vi "PIDSetpointSet.vi"(4 "Update":bool, 5 "Output Range":cluster{"output high":dbl, "output low":dbl}={"output high"=0.25, "output low"=-0.25}, 6 "Auto":bool, 7 "PID Gains":T1={"proportional gain (Kc)"=1.0, "integral time (Ti, min)"=0.01, "derivative time (Td, min)"=0.0}, 8 "Encoder Position":dbl format="%#_13g", 9 "Level":i8, 10 "Setpoints":dbl[](array[numeric]), 11 "Manual Power":dbl format="%#_13g") -> (0 "Power Out":dbl)   [LabVIEW 2018]
uses:
  <vilib>/addons/control/pid/pid.llb/PID (DBL).vi
  <vilib>/addons/control/pid/NI_PID_pid.lvlib
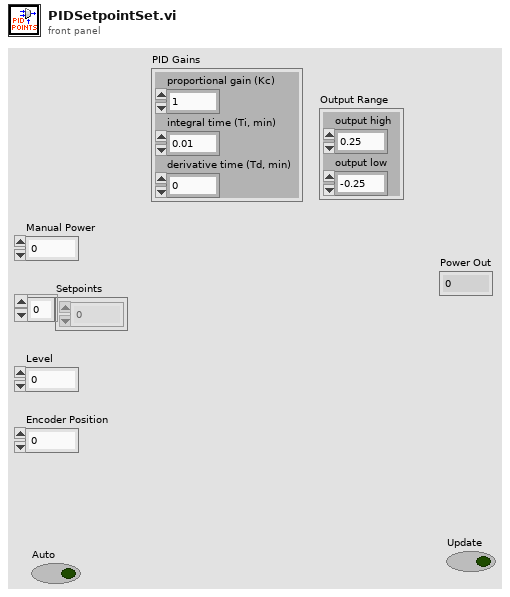
[diagram p1: front panel]
types:
  T1 = cluster{"proportional gain (Kc)":dbl, "integral time (Ti, min)":dbl, "derivative time (Td, min)":dbl}
  T2 = typedef "WPI_SwitchDevRef.ctl" = cluster{"DevStatus":errorcluster, "DIO Channel":T3, "CntIndex":T4, "Normally Closed":bool}
  T3 = typedef "FPGA_DIOChannel.ctl" = enum8{"DIO 0", "DIO 1", "DIO 2", "DIO 3", "DIO 4", "DIO 5", "DIO 6", "DIO 7", "DIO 8", "DIO 9", "DIO MXP 0", "DIO MXP 1", "DIO MXP 2", "DIO MXP 3", "DIO MXP 4", "DIO MXP 5", "DIO MXP 6", "DIO MXP 7", "DIO MXP 8", "DIO MXP 9", "DIO MXP 10", "DIO MXP 11", "DIO MXP 12", "DIO MXP 13", "DIO MXP 14", "DIO MXP 15", "SPI Port CS1", "SPI Port CS2", "SPI Port CS3", "SPI Port MISO", "SPI Port MOSI", "Invalid"}
  T4 = typedef "FPGA_CounterCtrSystemIndex.ctl" = enum8{"Ctr 0", "Ctr 1", "Ctr 2", "Ctr 3", "Ctr 4", "Ctr 5", "Ctr 6", "Ctr 7", "Invalid"}
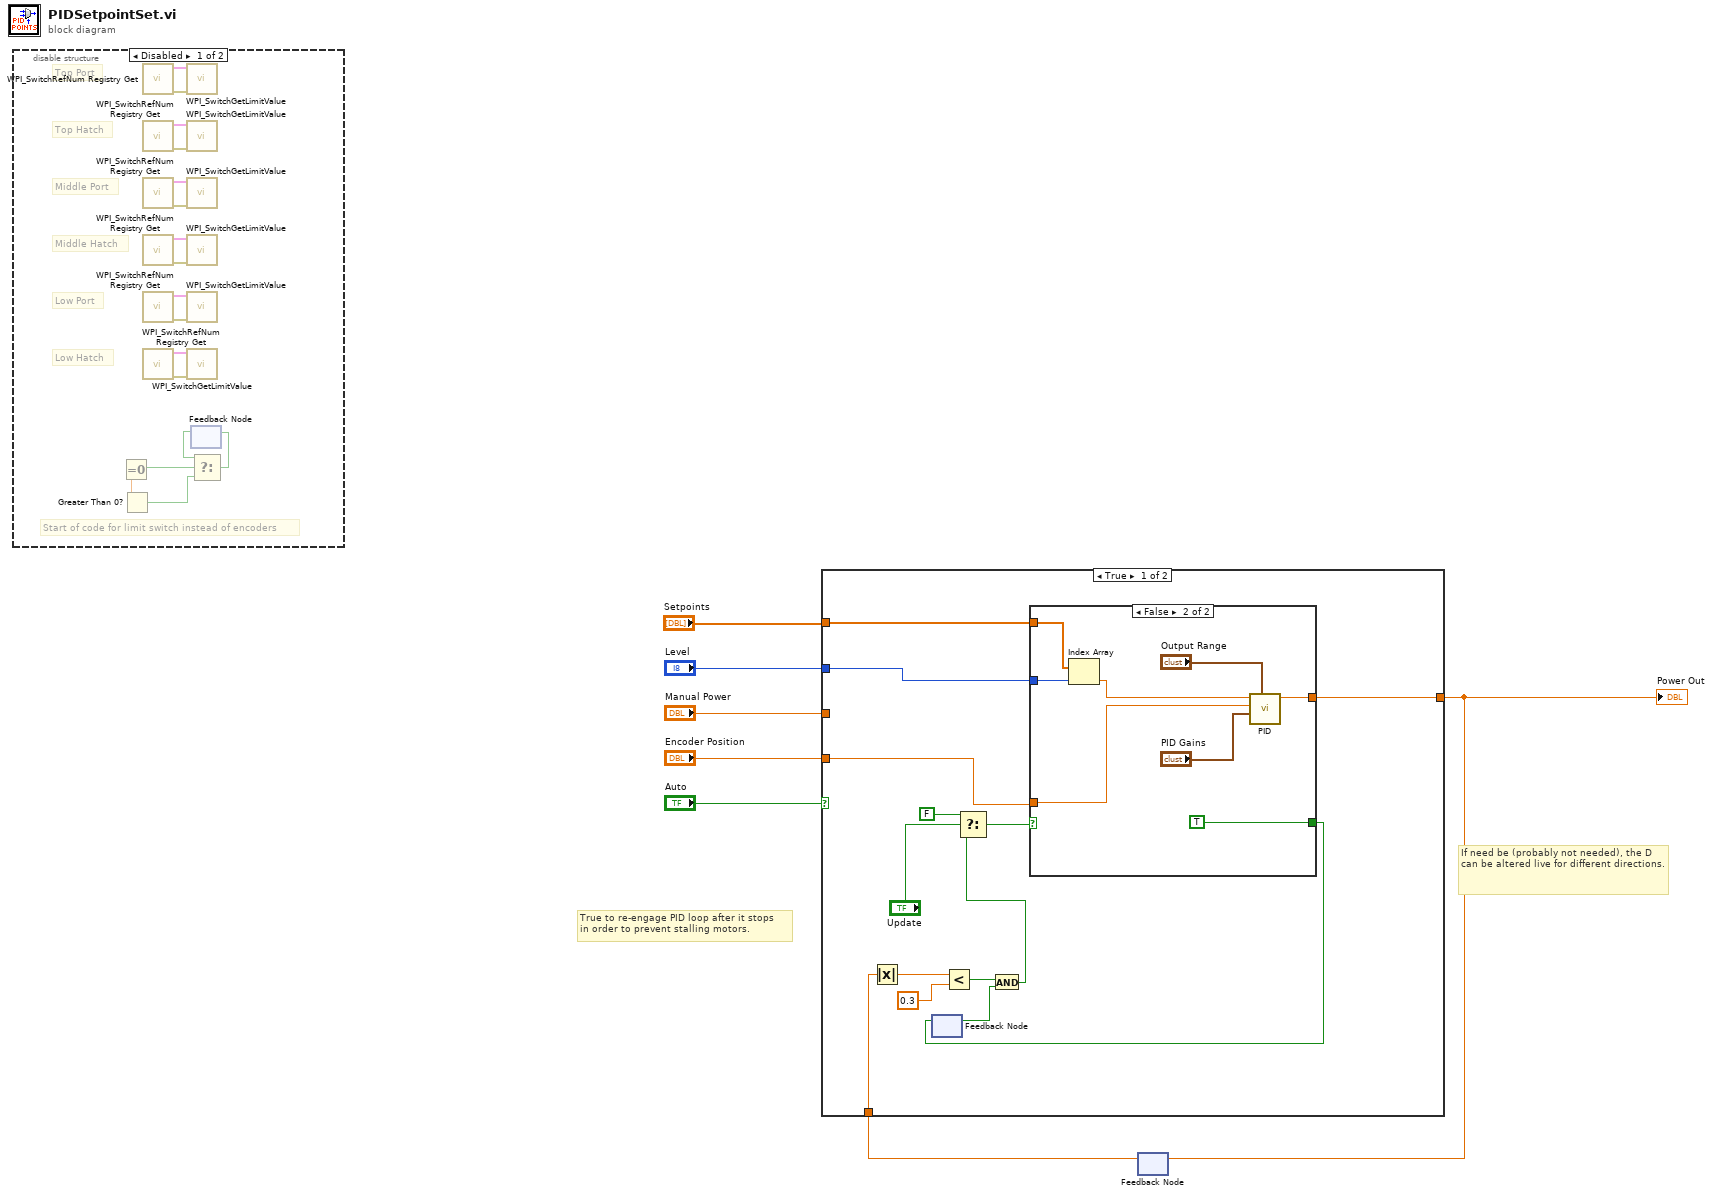
[diagram p0: block diagram]
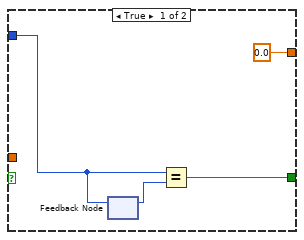
[diagram p3: hidden frame]
diagram:
  # "True to re-engage PID loop after it stops\nin order to prevent stalling motors."
  # "If need be (probably not needed), the D can be altered live for different directions."
  n1 = disable-structure shown="Disabled" {
    frame Disabled {
      # "Start of code for limit switch instead of encoders"
      # "Low Hatch"
      # "Low Port"
      # "Middle Hatch"
      # "Middle Port"
      # "Top Hatch"
      # "Top Port"
      n2 = Equal To 0?() -> (x=w8:dbl, x = 0?=w12:bool)
      n3 = Greater Than 0?(x=w8) -> (x > 0?=w11:bool)
      n4 = call <vilib>:"WPI_SwitchRefNum Registry Get.vi"() -> ("error out"=w24:errorcluster, "SwitchDevRef"=w23:T2)  [unwired: 10 in]
      n5 = call <vilib>:"WPI_SwitchRefNum Registry Get.vi"() -> ("error out"=w22:errorcluster, "SwitchDevRef"=w21:T2)  [unwired: 10 in]
      n6 = call <vilib>:"WPI_SwitchRefNum Registry Get.vi"() -> ("error out"=w20:errorcluster, "SwitchDevRef"=w19:T2)  [unwired: 10 in]
      n7 = call <vilib>:"WPI_SwitchRefNum Registry Get.vi"() -> ("error out"=w18:errorcluster, "SwitchDevRef"=w17:T2)  [unwired: 10 in]
      n8 = call <vilib>:"WPI_SwitchRefNum Registry Get.vi"() -> ("error out"=w16:errorcluster, "SwitchDevRef"=w15:T2)  [unwired: 10 in]
      n9 = call <vilib>:"WPI_SwitchRefNum Registry Get.vi"() -> ("error out"=w14:errorcluster, "SwitchDevRef"=w13:T2)  [unwired: 10 in]
      n10 = call <vilib>:"WPI_SwitchGetLimitValue.vi"("error in (no error)"=w24, "SwitchDevRef"=w23) -> ()  [unwired: 7 in, 3 out]
      n11 = call <vilib>:"WPI_SwitchGetLimitValue.vi"("error in (no error)"=w22, "SwitchDevRef"=w21) -> ()  [unwired: 7 in, 3 out]
      n12 = call <vilib>:"WPI_SwitchGetLimitValue.vi"("error in (no error)"=w20, "SwitchDevRef"=w19) -> ()  [unwired: 7 in, 3 out]
      n13 = call <vilib>:"WPI_SwitchGetLimitValue.vi"("error in (no error)"=w18, "SwitchDevRef"=w17) -> ()  [unwired: 7 in, 3 out]
      n14 = call <vilib>:"WPI_SwitchGetLimitValue.vi"("error in (no error)"=w16, "SwitchDevRef"=w15) -> ()  [unwired: 7 in, 3 out]
      n15 = call <vilib>:"WPI_SwitchGetLimitValue.vi"("error in (no error)"=w14, "SwitchDevRef"=w13) -> ()  [unwired: 7 in, 3 out]
      n16 = feedback #1() -> (w9:bool)  [unwired: 1 in]
      n17 = Select(t=w9, s=w12, f=w11) -> (s? t:f=w10:bool)
      n18 = feedback-in #1(w10) -> ()
    }
    frame Enabled {
    }
  }
  n19 = feedback #2() -> (w1:dbl)  [unwired: 1 in]
  n20 = case shown="True" "Auto" {
    tunnel: "Manual Power" -> [_ w51]
    tunnel: [w36 w51] -> w2
    tunnel: "Level" -> [w38 _]
    tunnel: "Setpoints" -> [w25 _]
    tunnel: "Encoder Position" -> [w37 _]
    tunnel: w1 -> [w27 _]
    frame True {
      n21 = Absolute Value(x=w27) -> (abs(x)=w26:dbl)
      n22 = feedback #3() -> (w33:bool)  [unwired: 1 in]
      n23 = Less?(x=w26, y=0.3) -> (x < y?=w34:bool)
      n24 = And(x=w34, y=w33) -> (x .and. y?=w30:bool)
      n25 = Select(t=FALSE, s="Update", f=w30) -> (s? t:f=w28:bool)
      n26 = case shown="False" w28 {
        tunnel: w38 -> [w41 w50]
        tunnel: w37 -> [_ w49]
        tunnel: [0.0 ("output") w46] -> w36
        tunnel: [w40 TRUE] -> w32
        tunnel: w25 -> [_ w44]
        frame True {
          n27 = feedback #4() -> (w42:i8)  [unwired: 1 in]
          n28 = feedback-in #4(w41) -> ()
          n29 = Equal?(x=w41, y=w42) -> (x = y?=w40:bool)
        }
        frame False {
          n30 = Index Array(array=w44, index=w50) -> (element=w43:dbl)
          n31 = call-poly <vilib>:"PID.vi"("output range"="Output Range", "PID gains"="PID Gains", "process variable"=w49, "setpoint"=w43) -> ("output"=w46:dbl)  [unwired: 6 in, 1 out]
        }
      }
      n32 = feedback-in #3(w32) -> ()
    }
    frame False {
    }
  }
  "Power Out" <- w2
  n33 = feedback-in #2(w2) -> ()
